vi "FG Default Authority.vi"(1 "FG Action (Read)":T1, 2 "Default Authority in":u8) -> (0 "Default Authority out":u8)   [LabVIEW 2009]
uses:
  cRIO/Functional Global Variables/Actions for FG's.ctl
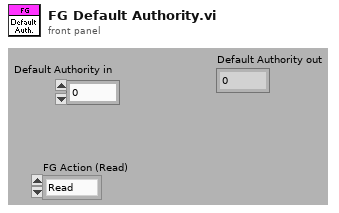
[diagram p1: front panel]
types:
  T1 = typedef "Actions for FG's.ctl" = enum16{"Read", "Write"}
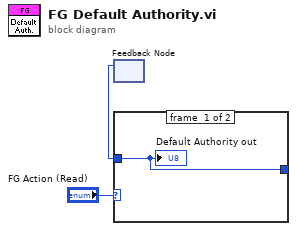
[diagram p0: block diagram]
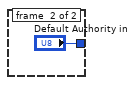
[diagram p2: hidden frame]
diagram:
  n1 = feedback #1() -> (w2:u8)  [unwired: 1 in]
  n2 = case shown="\"Read\", Default" "FG Action (Read)" {
    tunnel: w2 -> [w4 _]
    tunnel: [w4 "Default Authority in"] -> w3
    frame #0 {
      "Default Authority out" <- w4
    }
    frame #1 {
    }
  }
